vi "Update WeldCurrent in MeasDataQ.vi"(4 "UpdateTS (T)":bool=TRUE, 6 "TimeStamp":timestamp, 7 "AVCLockout":bool, 8 "error in (no error)":errorcluster, 9 "WeldCurrent":dbl, 11 "StepNumber":i32) -> (0 "error out":errorcluster, 3 "orData out":T1)   [LabVIEW 2017]
doc: "Developed by Kevin Thompson\nThompson Engineering, LLC\nkevin@thompsonengineering.net"
uses:
  TD MeasData QRef.ctl
  TD MeasData--cluster.ctl
  GBL DataQ Ref.vi
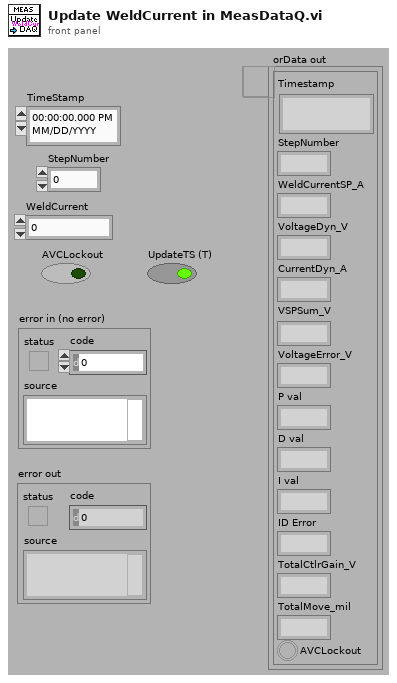
[diagram p1: front panel]
types:
  T1 = typedef "TD MeasData QRef.ctl" = refnum<queue>
  T2 = typedef "TD MeasData--cluster.ctl" = cluster{"Timestamp":timestamp, "StepNumber":i32, "WeldCurrentSP_A":dbl, "VoltageDyn_V":dbl, "CurrentDyn_A":dbl, "VSPSum_V":dbl, "VoltageError_V":dbl, "P val":dbl, "D val":dbl, "I val":dbl, "ID Error":dbl, "TotalCtlrGain_V":dbl, "TotalMove_mil":dbl, "AVCLockout":bool}
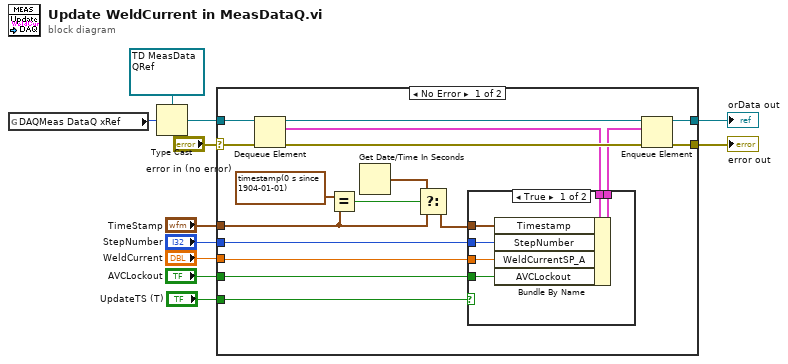
[diagram p0: block diagram]
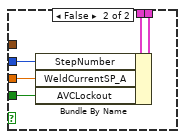
[diagram p2: hidden frame]
diagram:
  n1 = global read "GBL DataQ Ref.vi" "DAQMeas DataQ xRef"() -> (w5:u32)
  n2 = Type Cast(type=T1 refnum ("orData in"), x=w5) -> (*(type *) &x=w7:T1)
  n3 = case shown="No Error" "error in (no error)" {
    selector: "error in (no error)" -> [w23 w40]
    tunnel: w7 -> [w28 w41]
    tunnel: [w25 w40] -> w11
    tunnel: [w24 w41] -> w10
    tunnel: "TimeStamp" -> [w18 _]
    tunnel: "WeldCurrent" -> [w14 _]
    tunnel: "AVCLockout" -> [w15 _]
    tunnel: "StepNumber" -> [w13 _]
    tunnel: "UpdateTS (T)" -> [w12 _]
    frame No Error {
      n4 = Dequeue Element(queue=w28, error in (no error)=w23) -> (queue out=w26:T1, element=w22:T2, error out=w27:errorcluster)  [unwired: 1 in, 1 out]
      n5 = Equal?(x=timestamp(0 s since 1904-01-01) ("TimeStamp"), y=w18) -> (x = y?=w19:bool)
      n6 = Get Date/Time In Seconds() -> (seconds since 1Jan1904=w16:timestamp)
      n7 = Select(t=w16, s=w19, f=w18) -> (s? t:f=w17:timestamp)
      n8 = case shown="True" w12 {
        tunnel: w22 -> [w34 w39]
        tunnel: [w33 w38] -> w21
        tunnel: w17 -> [w32 _]
        tunnel: w15 -> [w31 w37]
        tunnel: w14 -> [w30 w36]
        tunnel: w13 -> [w29 w35]
        frame True {
          n9 = Bundle By Name(cluster=w34, "Timestamp"=w32, "StepNumber"=w29, "WeldCurrentSP_A"=w30, "AVCLockout"=w31) -> (w33:T2)
        }
        frame False {
          n10 = Bundle By Name(cluster=w39, "StepNumber"=w35, "WeldCurrentSP_A"=w36, "AVCLockout"=w37) -> (w38:T2)
        }
      }
      n11 = Enqueue Element(queue=w26, element=w21, error in (no error)=w27) -> (queue out=w24:T1, error out=w25:errorcluster)  [unwired: 1 in, 1 out]
    }
    frame Error {
    }
  }
  "orData out" <- w10
  "error out" <- w11
